vi "img test14(coutsegment attempt3).vi"() -> ()   [LabVIEW 2014]
uses:
  <vilib>/vision/NI_Vision_Development_Module.lvlib
panel:
  out "Array":dbl[][](array[numeric])
  in  "fast forward":bool
  out "Bottom Full movement patterns":string[](array[string])
  out "Top Full movement patterns":string[](array[string])
  out "bottom player pattern count 2":i32[](array[numeric])
  out "bottom player patterns 2":string[](array[string])
  out "top player pattern count":i32[](array[numeric])
  out "Top player patterns":string[](array[string])
  out "start":i32[](array[numeric])
  out "end":i32[](array[numeric])
  out "Infered action indicators":string[][](array[string])
  out "Movement data from both players":i32[][](array[numeric])
  out "end":i32[](array[numeric])
  out "start":i32[](array[numeric])
  in  "start":bool
  in  "End":bool
  in  "output array 4":string[][](array[string])
  in  "output array 3":string[][](array[string])
  in  "output array 2":string[][](array[string])=array2129x6[12774 elements]
  out "BOTTOM":string[](array[string])
  out "TOP":string[](array[string])
  in  "output array":string[][](array[string])=array1935x6[11610 elements]
  out "Number of Frames":u32
  out "Top player court segment display 2":bool[][](array[boolean])
  out "count top":i32[](graph)
  out "count bottom":i32[](graph)
  out "trans top":i32[](graph)
  out "trans bottom":i32[](graph)
  in  "ON":bool
  out "Top player court segment display":bool[][](array[boolean])
  out "bottom player":cluster{"Numeric":dbl, "Numeric":dbl}[](array[cluster])
  out "top player":cluster{"Numeric":dbl, "Numeric":dbl}[](array[cluster])
  in  "playing":bool
  out "Top VIew":cluster{"Numeric":dbl, "Numeric":dbl}[](graph)
  out "Image 4":T1(plugin-control)
  in  "frame jump":i32=3
  in  "speed":u32(slide)
  in  "start":i32(slide) step=219843704 scale=0.0..66731.0
  out "Image 3":T1(plugin-control)
  in  "AVI Path":path=path "E:/PhD work/PhD research work/Videos/Chen Jin vs Hu Yun (Edited).avi"
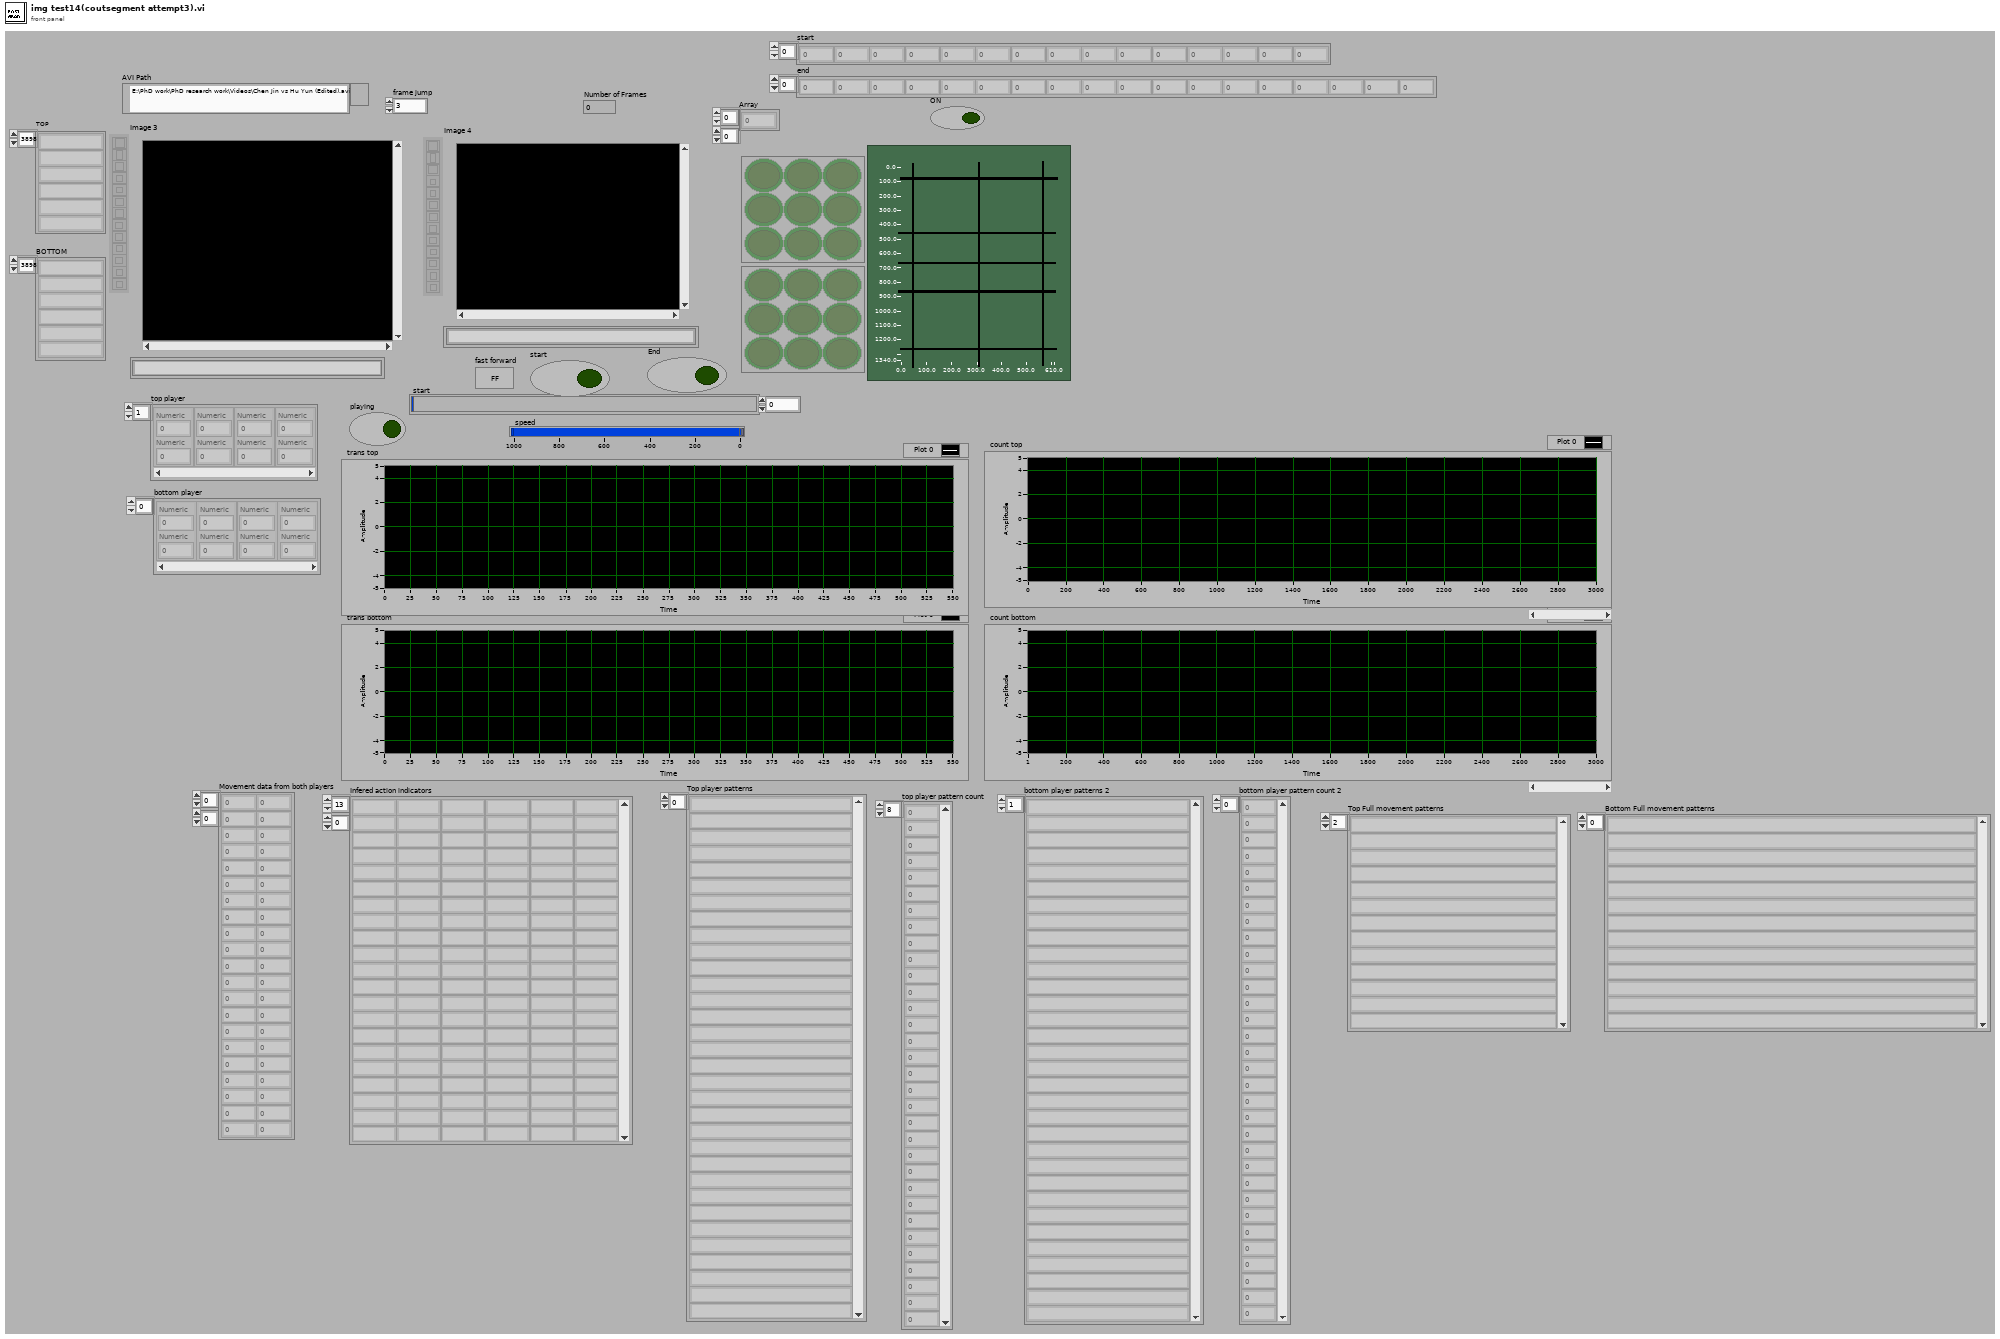
[diagram p1: front panel]
types:
  T1 = typedef "IMAQ Image.ctl" = refnum<image>
  T2 = cluster{cluster{"X":sgl, "Y":sgl}[], cluster{i32, i32}[], "Unit":u32}
  T3 = typedef "Image Type" = u32
  T4 = typedef "AviRefnum.ctl" = refnum<k1>
  T5 = cluster{"width":u32, "height":u32, "framesPerSecond":u32, "compressionFilter":string, "hasData":bool}
  T6 = cluster{"Origin Pixel":cluster{"X":sgl, "Y":sgl}, "Angle Relative to Horizontal (deg)":sgl, "Axis Reference":u32}
  T7 = typedef "Particle Parameters" = i32
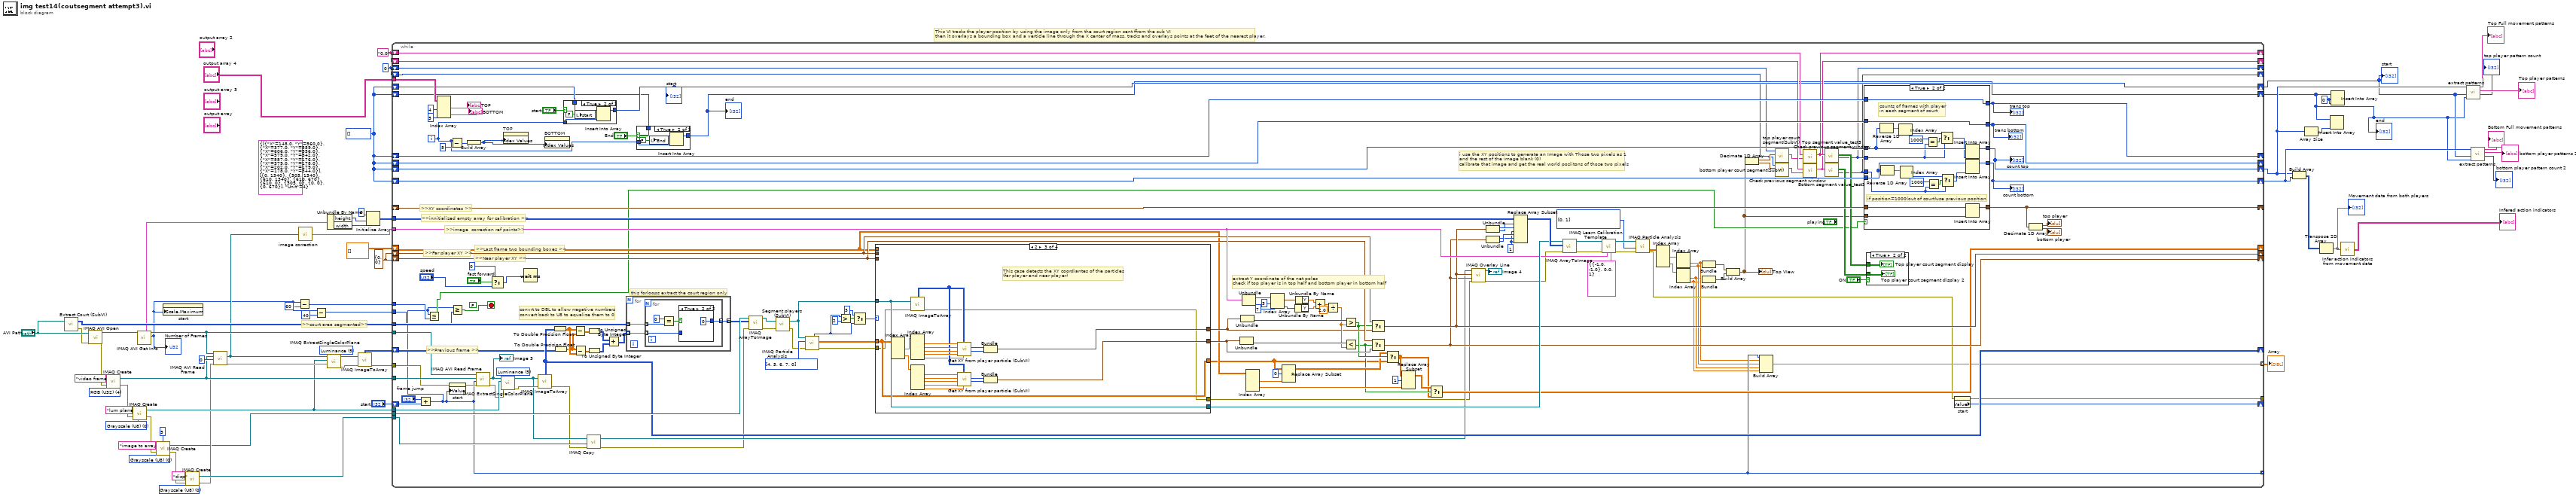
[diagram p0: block diagram]
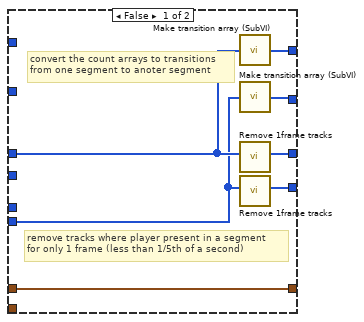
[diagram p4: hidden frame]
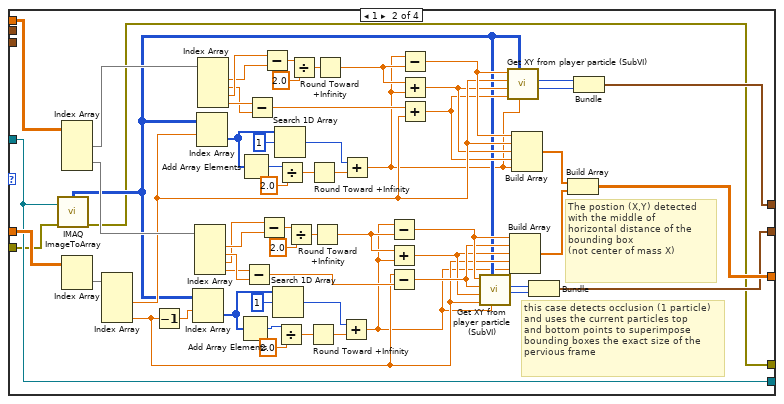
[diagram p7: hidden frame]
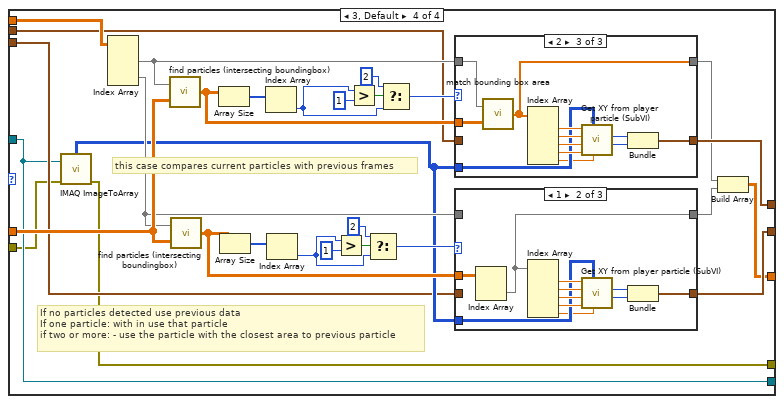
[diagram p8: hidden frame]
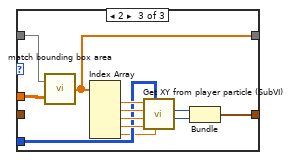
[diagram p10: hidden frame]
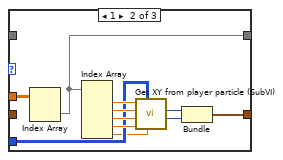
[diagram p12: hidden frame]
diagram:
  w2 = 0 ("Top player segment value")
  w14 = 0 ("index")
  (unwired) T2 {[{"X"=148.0, "Y"=560.0}, {"X"=377.0, "Y"=559.0}, {"X"=606.0, "Y"=556.0}, {"X"=579.0, "Y"=342.0}, {"X"=557.0, "Y"=176.0}, {"X"=379.0, "Y"=178.0}, {"X"=202.0, "Y"=179.0}, {"X"=178.0, "Y"=344.0}], [{0, 1340}, {305, 1340}, {610, 1340}, {610, 670}, {610, 0}, {305, 0}, {0, 0}, {0, 670}], "Unit"=4} ("ref points")
  w27 = "0,0" ("Player segment position")
  w18 = i32[] [] ("input array")
  w37 = cluster{"X coordinate":i32, "Y coordinate":i32} {"X coordinate"=0, "Y coordinate"=0}
  w50 = T3 0 items=["Grayscale (U8)", "Grayscale (I16)", "Grayscale (SGL)", "Complex (CSG)", "RGB (U32)", "HSL (U32)", "RGB (U64)", "Grayscale (U16)"] ("Image Type")
  w57 = 5 items=["Red", "Green", "Blue", "Hue", "Saturation", "Luminance", "Value", "Intensity"] ("Color Plane")
  w58 = T3 0 items=["Grayscale (U8)", "Grayscale (I16)", "Grayscale (SGL)", "Complex (CSG)", "RGB (U32)", "HSL (U32)", "RGB (U64)", "Grayscale (U16)"] ("Image Type")
  w62 = T3 0 items=["Grayscale (U8)", "Grayscale (I16)", "Grayscale (SGL)", "Complex (CSG)", "RGB (U32)", "HSL (U32)", "RGB (U64)", "Grayscale (U16)"] ("Image Type")
  w60 = T3 4 items=["Grayscale (U8)", "Grayscale (I16)", "Grayscale (SGL)", "Complex (CSG)", "RGB (U32)", "HSL (U32)", "RGB (U64)", "Grayscale (U16)"] ("Image Type")
  # ">>court area segmented>>"
  # "This VI tracks the player position by using the image only from the court region sent ffrom the sub VI\nthen it overlays a bounding box and a verticle line through the X center of mass. tracks and overlays points at the feet of the nearest player."
  n1 = call "Extract Court (SubVI).vi"("AVI Path"="AVI Path") -> ("error out"=w64:errorcluster, "Court pixels out"=w40:u8[][])  [unwired: 1 in]
  n2 = call "IMAQ AVI Open"("error in (no error)"=w64, "AVI Path"="AVI Path") -> ("error out"=w46:errorcluster, "Avi Refnum"=w35:T4)  [unwired: 8 in]
  n3 = call "IMAQ Create"("Image Name"="video frame", "Image Type"=w60, "error in (no error)"=w46) -> ("New Image"=w54:T1, "error out"=w45:errorcluster)  [unwired: 2 in]
  n4 = call "IMAQ Create"("Image Name"="lum plane", "Image Type"=w62, "error in (no error)"=w45) -> ("New Image"=w53:T1, "error out"=w44:errorcluster)  [unwired: 2 in]
  n5 = call "IMAQ AVI Get Info"("Avi Refnum"=w35) -> ("Number of Frames"=w25:u32, "Avi Refnum (duplicate)"=w34:T4, "Frame Data"=w31:T5)  [unwired: 6 in, 2 out]
  "Number of Frames" <- w25
  n6 = call "IMAQ Create"("Border Size"=5, "Image Name"="image to array", "Image Type"=w58, "error in (no error)"=w44) -> ("New Image"=w39:T1, "error out"=w43:errorcluster)  [unwired: 1 in]
  n7 = property on="start" class="Slide (strict)"("Scale.Maximum"=w25) -> ()  [unwired: 2 in, 2 out]
  n8 = call "IMAQ Create"("Image Name"="disp", "Image Type"=w50, "error in (no error)"=w43) -> ("New Image"=w48:T1, "error out"=w42:errorcluster)  [unwired: 2 in]
  n9 = call "IMAQ AVI Read Frame"("error in (no error)"=w42, "Frame Number"=u32 0, "Image"=w54, "Avi Refnum"=w34) -> ("error out"=w56:errorcluster, "Image Out"=w26:T1)  [unwired: 4 in, 2 out]
  n10 = Subtract(x=w25, y=u32 60) -> (x-y=w22:u32)
  n11 = call "image correction.vi"("Image"=w26) -> ("ref points"=w20:T2)
  n12 = Subtract(x=w25, y=u32 40) -> (x-y=w21:u32)
  n13 = Unbundle By Name(w31) -> ("height"=w30:u32, "width"=w29:u32)
  n14 = call "IMAQ ExtractSingleColorPlane"("Color Plane"=w57, "error in (no error)"=w56, "Image Dst"=w53, "Image Src"=w26) -> ("error out"=w47:errorcluster, "Image Dst Out"=w51:T1)  [unwired: 6 in]
  n15 = call "IMAQ ImageToArray"("error in (no error)"=w47, "Image"=w51) -> ("error out"=w33:errorcluster, "Image Pixels (U8)"=w52:u8[][])  [unwired: 2 in, 3 out]
  n16 = Initialize Array(u8 0 ("element"), w30, w29) -> (w28:u8[][])
  n17 = while {
    tunnel: w34 -> [w187]
    tunnel: w54 -> [w204]
    tunnel: w40 -> [w217]
    tunnel: w53 -> [w205]
    tunnel: w39 -> [w216]
    shift-right: [w215] -> _
    shift-left: w52 -> [w214]
    tunnel: w48 -> [w190]
    shift-right: [w133] -> _
    shift-left: dbl[][] [] ("Particle Measurements (Pixels)") -> [w143]
    shift-right: [w147] -> _
    shift-left: w37 -> [w149]
    shift-right: [w145] -> _
    shift-left: w37 -> [w148]
    shift-right: [w184] -> _
    shift-left: "start" -> [w189]
    tunnel: w33 -> [w186]
    tunnel: w28 -> [w183]
    tunnel: w20 -> [w162]
    shift-right: [w117] -> _
    shift-left: _ -> [w166]
    shift-right: [w92] -> w12
    shift-left: w18 -> [w120]
    shift-right: [w93] -> w11
    shift-left: w18 -> [w121]
    tunnel: [w123] -> _
    shift-right: [w111] -> _
    shift-left: w18 -> [w118]
    shift-right: [w116] -> _
    shift-left: w18 -> [w119]
    shift-right: [w105] -> _
    shift-left: w27 -> [w112]
    shift-right: [w106] -> _
    shift-left: w27 -> [w113]
    tunnel: w22 -> [w104]
    tunnel: w21 -> [w103]
    tunnel: [w71] -> _ mode=indexing
    tunnel: "output array 4" -> [w98]
    shift-right: [w84] -> w3
    shift-left: w18 -> [w85]
    shift-right: [w86] -> w4
    shift-left: w18 -> [w87]
    shift-right: [w75] -> _
    shift-left: w2 -> [w73]
    shift-right: [w74] -> _
    shift-left: w2 -> [w72]
    tunnel: [w66] -> w1 mode=indexing
    i -> [w82]
    stop <- w110 stop-if-true
    w170 = T7[] [0, 1] items=["Center of Mass X", "Center of Mass Y", "First Pixel X", "First Pixel Y", "Bounding Rect Left", "Bounding Rect Top", "Bounding Rect Right", "Bounding Rect Bottom", "Max Feret Diameter Start X", "Max Feret Diameter Start Y", "Max Feret Diameter End X", "Max Feret Diameter End Y", "Max Horiz. Segment Length Left", "Max Horiz. Segment Length Right", "Max Horiz. Segment Length Row", "-", "Bounding Rect Width", "Bounding Rect Height", "Bounding Rect Diagonal", "Perimeter", "Convex Hull Perimeter", "Holes' Perimeter", "Max Feret Diameter", "Equivalent Ellipse Major Axis", "Equivalent Ellipse Minor Axis", "Equivalent Ellipse Minor Axis (Feret)", "Equivalent Rect Long Side", "Equivalent Rect Short Side", "Equivalent Rect Diagonal", "Equivalent Rect Short Side (Feret)", "Average Horiz. Segment Length", "Average Vert. Segment Length", "Hydraulic Radius", "Waddel Disk Diameter", "-", "Area", "Holes' Area", "Particle & Holes' Area", "Convex Hull Area", "Image Area", "-", "Number of Holes", "Number of Horiz. Segments", "Number of Vert. Segments", "-", "Orientation", "Max Feret Diameter Orientation", "-", "% Area/Image Area", "% Area/(Particle & Holes' Area)", "Ratio of Equivalent Ellipse Axes", "Ratio of Equivalent Rect Sides", "-", "Elongation Factor", "Compactness Factor", "Heywood Circularity Factor", "Type Factor", "-", "Sum X", "Sum Y", "Sum XX", "Sum XY", "Sum YY", "Sum XXX", "Sum XXY", "Sum XYY", "Sum YYY", "-", "Moment of Inertia XX", "Moment of Inertia XY", "Moment of Inertia YY", "Moment of Inertia XXX", "Moment of Inertia XXY", "Moment of Inertia XYY", "Moment of Inertia YYY", "Norm. Moment of Inertia XX", "Norm. Moment of Inertia XY", "Norm. Moment of Inertia YY", "Norm. Moment of Inertia XXX", "Norm. Moment of Inertia XXY", "Norm. Moment of Inertia XYY", "Norm. Moment of Inertia YYY", "Hu Moment 1", "Hu Moment 2", "Hu Moment 3", "Hu Moment 4", "Hu Moment 5", "Hu Moment 6", "Hu Moment 7"] ("Real-World Measurements")
    w178 = u8 1 ("new element/subarray")
    w206 = T7[] [4, 5, 6, 7, 0] items=["Center of Mass X", "Center of Mass Y", "First Pixel X", "First Pixel Y", "Bounding Rect Left", "Bounding Rect Top", "Bounding Rect Right", "Bounding Rect Bottom", "Max Feret Diameter Start X", "Max Feret Diameter Start Y", "Max Feret Diameter End X", "Max Feret Diameter End Y", "Max Horiz. Segment Length Left", "Max Horiz. Segment Length Right", "Max Horiz. Segment Length Row", "-", "Bounding Rect Width", "Bounding Rect Height", "Bounding Rect Diagonal", "Perimeter", "Convex Hull Perimeter", "Holes' Perimeter", "Max Feret Diameter", "Equivalent Ellipse Major Axis", "Equivalent Ellipse Minor Axis", "Equivalent Ellipse Minor Axis (Feret)", "Equivalent Rect Long Side", "Equivalent Rect Short Side", "Equivalent Rect Diagonal", "Equivalent Rect Short Side (Feret)", "Average Horiz. Segment Length", "Average Vert. Segment Length", "Hydraulic Radius", "Waddel Disk Diameter", "-", "Area", "Holes' Area", "Particle & Holes' Area", "Convex Hull Area", "Image Area", "-", "Number of Holes", "Number of Horiz. Segments", "Number of Vert. Segments", "-", "Orientation", "Max Feret Diameter Orientation", "-", "% Area/Image Area", "% Area/(Particle & Holes' Area)", "Ratio of Equivalent Ellipse Axes", "Ratio of Equivalent Rect Sides", "-", "Elongation Factor", "Compactness Factor", "Heywood Circularity Factor", "Type Factor", "-", "Sum X", "Sum Y", "Sum XX", "Sum XY", "Sum YY", "Sum XXX", "Sum XXY", "Sum XYY", "Sum YYY", "-", "Moment of Inertia XX", "Moment of Inertia XY", "Moment of Inertia YY", "Moment of Inertia XXX", "Moment of Inertia XXY", "Moment of Inertia XYY", "Moment of Inertia YYY", "Norm. Moment of Inertia XX", "Norm. Moment of Inertia XY", "Norm. Moment of Inertia YY", "Norm. Moment of Inertia XXX", "Norm. Moment of Inertia XXY", "Norm. Moment of Inertia XYY", "Norm. Moment of Inertia YYY", "Hu Moment 1", "Hu Moment 2", "Hu Moment 3", "Hu Moment 4", "Hu Moment 5", "Hu Moment 6", "Hu Moment 7"] ("Pixel Measurements")
    (unwired) FALSE
    w218 = 5 items=["Red", "Green", "Blue", "Hue", "Saturation", "Luminance", "Value", "Intensity"] ("Color Plane")
    # ">>XY coordinates >>"
    # ">>innitialized empty array for calibration >>"
    # ">>image  correction ref points>>"
    # "extract Y coordinate of the net poles\ncheck if top player is in top half and bottom player in bottom half"
    # "i use the XY positions to generate an Image with Those two pixels as 1 \nand the rest of the image blank (0)\ncalibrate that image and get the real world posiitons of those two pixels"
    # ">>Last frame two bounding boxes >>"
    # ">>Far player XY >>"
    # ">>Near player XY >>"
    # ">>Previous frame >>"
    # "convrt to DBL to allow negative numbers\nconvert back to U8 to equalize them to 0"
    # "this forloops extract the court region only"
    n18 = Add(x="frame jump", y=w189) -> (x+y=w71:i32)
    n19 = Less Or Equal?(x=w71, y=w104) -> (x <= y?=w109:bool)
    n20 = Index Array(array=w98, index (col) #1=4 ("disabled index (col)"), index (col) #2=5 ("index (col)")) -> (element #1=→"TOP":string[], element #2=→"BOTTOM":string[])  [unwired: 2 in]
    n21 = property on="start" class="Slide (strict)"(error in=w186, "Value"=w71) -> (error out=w185:errorcluster)  [unwired: 1 in, 1 out]
    n22 = Subtract(x=w82, y=5) -> (x-y=w90:i32)
    n23 = Greater Or Equal?(x=w71, y=w103) -> (x >= y?=w110:bool)
    n24 = Build Array(w90) -> (w89:i32[])
    n25 = call "IMAQ AVI Read Frame"("error in (no error)"=w185, "Frame Number"=w71, "Image"=w204, "Avi Refnum"=w187) -> ("error out"=w99:errorcluster, "Image Out"=w102:T1)  [unwired: 4 in, 2 out]
    "Image 3" <- w102
    n26 = Select(t=u32 0, s="fast forward", f="speed") -> (s? t:f=w77:u32)
    n27 = call "IMAQ ExtractSingleColorPlane"("Color Plane"=w218, "error in (no error)"=w99, "Image Dst"=w205, "Image Src"=w102) -> ("error out"=w207:errorcluster, "Image Dst Out"=w191:T1)  [unwired: 6 in]
    n28 = property on="TOP" class="Arr (strict)"("Index Values"=w89) -> ()  [unwired: 2 in, 2 out]
    n29 = Wait (ms)(milliseconds to wait=w77) -> ()  [unwired: 1 out]
    n30 = call "IMAQ ImageToArray"("error in (no error)"=w207, "Image"=w191) -> ("error out"=w128:errorcluster, "Image Pixels (U8)"=w215:u8[][])  [unwired: 2 in, 3 out]
    n31 = property on="BOTTOM" class="Arr (strict)"("Index Values"=w89) -> ()  [unwired: 2 in, 2 out]
    n32 = To Double Precision Float(number=w215) -> (double precision float=w211:dbl[][])
    n33 = To Double Precision Float(number=w214) -> (double precision float=w210:dbl[][])
    n34 = case shown="True" "start" {
      tunnel: w87 -> [w224 w228]
      tunnel: w82 -> [_ w227]
      tunnel: [w224 w226] -> w86
      frame False {
      }
      frame True {
        n35 = local write "start"(FALSE ("start")) -> ()
        n36 = Insert Into Array(array=w228, new element=w227) -> (w226:i32[])  [unwired: 1 in]
      }
    }
    "start" <- w86
    n37 = Subtract(x=w211, y=w210) -> (x-y=w209:dbl[][])
    n38 = Subtract(x=w210, y=w211) -> (x-y=w208:dbl[][])
    n39 = call "IMAQ Copy"("error in (no error)"=w128, "Image Dst"=w190, "Image Src"=w191) -> ("error out"=w127:errorcluster, "Image Dst Out"=w129:T1)  [unwired: 3 in]
    n40 = To Unsigned Byte Integer(number=w209) -> (unsigned 8bit integer=w213:u8[][])
    n41 = To Unsigned Byte Integer(number=w208) -> (unsigned 8bit integer=w212:u8[][])
    n42 = Add(x=w213, y=w212) -> (x+y=w81:u8[][])
    n43 = for {
      tunnel: w217 -> [w429] mode=indexing
      tunnel: [w428] -> w80 mode=indexing
      tunnel: w81 -> [w427] mode=indexing
      n44 = for {
        tunnel: w429 -> [w434] mode=indexing
        tunnel: [w431] -> w428 mode=indexing
        tunnel: w427 -> [w430] mode=indexing
        n45 = Equal?(x=u8 0, y=w434) -> (x = y?=w432:bool)
        n46 = case shown="True" w432 {
          tunnel: [w435 u8 0 ("x")] -> w431
          tunnel: w430 -> [w435 _]
          frame False {
          }
          frame True {
          }
        }
      }
    }
    n47 = case shown="True" "End" {
      tunnel: w85 -> [w219 w223]
      tunnel: w82 -> [_ w222]
      tunnel: [w219 w221] -> w84
      frame False {
      }
      frame True {
        n48 = local write "End"(FALSE ("End")) -> ()
        n49 = Insert Into Array(array=w223, new element=w222) -> (w221:i32[])  [unwired: 1 in]
      }
    }
    "end" <- w84
    n50 = call "IMAQ ArrayToImage"("error in (no error)"=w127, "Image Pixels (U8)"=w80, "Image"=w216) -> ("error out"=w202:errorcluster, "Image Out"=w203:T1)  [unwired: 7 in]
    n51 = call "Segment players (SubVI).vi"("error In"=w202, "Image In"=w203) -> ("error out"=w196:errorcluster, "Image Out"=w194:T1)
    n52 = call "IMAQ Particle Analysis"("error in (no error)"=w196, "Pixel Measurements"=w206, "Image"=w194) -> ("error out"=w195:errorcluster, "Particle Measurements (Pixels)"=w193:dbl[][], "Number of Particles"=w198:i32)  [unwired: 3 in, 3 out]
    n53 = Greater?(x=w198, y=2) -> (0:w201:bool)
    n54 = Select(t=3 ("y"), s=w201, f=w198) -> (s? t:f=w197:i32)
    n55 = case shown="2" w197 {
      tunnel: [w262 w289 w343 w353] -> w176
      tunnel: w193 -> [_ w324 w329 w373]
      tunnel: w195 -> [w259 w265 w326 w349]
      tunnel: w194 -> [w262 w289 w343 w353]
      tunnel: [w260 w273 w331 w355] -> w144
      tunnel: [w261 w280 w330 w354] -> w146
      tunnel: [w263 w290 w329 w350] -> w132
      tunnel: w143 -> [w263 w314 _ w376]
      tunnel: w149 -> [w261 _ _ w361]
      tunnel: w148 -> [w260 _ _ w356]
      tunnel: [w259 w264 w325 w348] -> w125
      frame 0 {
        # "This case identifies frames where no particles are detected and keeps the same values from the\nprevious frame"
      }
      frame 1 {
        # "The postion (X,Y) detected with the middle of \nhorizontal distance of the bounding box\n(not center of mass X)"
        # "this case detects occlusion (1 particle)\nand uses the current particles top \nand bottom points to superimpose \nbounding boxes the exact size of the \npervious frame"
        n56 = call "IMAQ ImageToArray"("error in (no error)"=w265, "Image"=w289) -> ("error out"=w264:errorcluster, "Image Pixels (U8)"=w272:u8[][])  [unwired: 2 in, 3 out]
        n57 = Index Array(array=w314) -> (element #1=w322:dbl[], element #2=w294:dbl[])  [unwired: 4 in]
        n58 = Index Array(array=w324) -> (element=w323:dbl[])  [unwired: 2 in]
        n59 = Index Array(array=w323) -> (element #2=w285:dbl, element #4=w276:dbl)  [unwired: 4 in, 2 out]
        n60 = Decrement(x=w276) -> (x-1=w287:dbl)
        n61 = Index Array(array=w272, index (row)=w287) -> (element=w309:u8[])  [unwired: 1 in]
        n62 = Index Array(array=w294) -> (element #1=w298:dbl, element #2=w301:dbl, element #3=w297:dbl, element #4=w300:dbl)  [unwired: 4 in]
        n63 = Index Array(array=w272, index (row)=w285) -> (element=w302:u8[])  [unwired: 1 in]
        n64 = Index Array(array=w322) -> (element #1=w318:dbl, element #2=w315:dbl, element #3=w319:dbl, element #4=w316:dbl)  [unwired: 4 in]
        n65 = Add Array Elements(numeric array=w309) -> (sum=w310:u8)
        n66 = Add Array Elements(numeric array=w302) -> (sum=w306:u8)
        n67 = Subtract(x=w300, y=w301) -> (x-y=w288:dbl)
        n68 = Subtract(x=w316, y=w315) -> (x-y=w293:dbl)
        n69 = Subtract(x=w297, y=w298) -> (x-y=w296:dbl)
        n70 = Subtract(x=w319, y=w318) -> (x-y=w320:dbl)
        n71 = Search 1D Array(1D array=w309, element=u8 1) -> (index of element=w308:i32)  [unwired: 1 in]
        n72 = Search 1D Array(1D array=w302, element=u8 1) -> (index of element=w307:i32)  [unwired: 1 in]
        n73 = Divide(x=w310, y=2.0) -> (x/y=w311:dbl)
        n74 = Divide(x=w306, y=2.0) -> (x/y=w305:dbl)
        n75 = Divide(x=w296, y=2.0) -> (x/y=w299:dbl)
        n76 = Divide(x=w320, y=2.0) -> (x/y=w317:dbl)
        n77 = Round Toward +Infinity(x=w311) -> (ceil(x): smallest int >= x=w270:dbl)
        n78 = Round Toward +Infinity(x=w305) -> (ceil(x): smallest int >= x=w269:dbl)
        n79 = Round Toward +Infinity(x=w299) -> (ceil(x): smallest int >= x=w271:dbl)
        n80 = Round Toward +Infinity(x=w317) -> (ceil(x): smallest int >= x=w268:dbl)
        n81 = Add(x=w308, y=w270) -> (x+y=w266:dbl)
        n82 = Add(x=w307, y=w269) -> (x+y=w267:dbl)
        n83 = Subtract(x=w266, y=w271) -> (x-y=w279:dbl)
        n84 = Add(x=w271, y=w266) -> (x+y=w277:dbl)
        n85 = Subtract(x=w276, y=w288) -> (x-y=w278:dbl)
        n86 = Subtract(x=w267, y=w268) -> (x-y=w286:dbl)
        n87 = Add(x=w268, y=w267) -> (x+y=w284:dbl)
        n88 = Add(x=w293, y=w285) -> (x+y=w283:dbl)
        n89 = call "Get XY from player particle (SubVI).vi"("Center of mass X"=w266, "Image in Pixels (U8)"=w272, "Particle bounding rect bottom"=w276, "Particle bounding rect right"=w277, "Particle bounding rect top"=w278, "Particle bounding rect left"=w279) -> ("Y coordinate"=w274:i32, "X coordinate"=w275:i32)  [unwired: 2 in]
        n90 = call "Get XY from player particle (SubVI).vi"("Center of mass X"=w267, "Image in Pixels (U8)"=w272, "Particle bounding rect bottom"=w283, "Particle bounding rect right"=w284, "Particle bounding rect top"=w285, "Particle bounding rect left"=w286) -> ("Y coordinate"=w281:i32, "X coordinate"=w282:i32)  [unwired: 2 in]
        n91 = Build Array(w279, w278, w277, w276, w266) -> (w291:dbl[])
        n92 = Build Array(w286, w285, w284, w283, w267) -> (w292:dbl[])
        n93 = Bundle("X coordinate"=w275, "Y coordinate"=w274) -> (w273:cluster{"X coordinate":i32, "Y coordinate":i32})  [unwired: 1 in]
        n94 = Build Array(w292, w291) -> (w290:dbl[][])
        n95 = Bundle("X coordinate"=w282, "Y coordinate"=w281) -> (w280:cluster{"X coordinate":i32, "Y coordinate":i32})  [unwired: 1 in]
      }
      frame 2 {
        # "This case detects the XY coordiantes of the particles\n(far player and near player)"
        n96 = Index Array(array=w329) -> (element #1=w337:dbl[], element #2=w336:dbl[])  [unwired: 4 in]
        n97 = call "IMAQ ImageToArray"("error in (no error)"=w326, "Image"=w343) -> ("error out"=w325:errorcluster, "Image Pixels (U8)"=w338:u8[][])  [unwired: 2 in, 3 out]
        n98 = Index Array(array=w337) -> (element #1=w347:dbl, element #2=w346:dbl, element #3=w345:dbl, element #4=w344:dbl, element #5=w328:dbl)  [unwired: 5 in]
        n99 = Index Array(array=w336) -> (element #1=w339:dbl, element #2=w340:dbl, element #3=w341:dbl, element #4=w342:dbl, element #5=w327:dbl)  [unwired: 5 in]
        n100 = call "Get XY from player particle (SubVI).vi"("Center of mass X"=w328, "Image in Pixels (U8)"=w338, "Particle bounding rect bottom"=w344, "Particle bounding rect right"=w345, "Particle bounding rect top"=w346, "Particle bounding rect left"=w347) -> ("Y coordinate"=w334:i32, "X coordinate"=w335:i32)  [unwired: 2 in]
        n101 = call "Get XY from player particle (SubVI).vi"("Center of mass X"=w327, "Image in Pixels (U8)"=w338, "Particle bounding rect bottom"=w342, "Particle bounding rect right"=w341, "Particle bounding rect top"=w340, "Particle bounding rect left"=w339) -> ("Y coordinate"=w332:i32, "X coordinate"=w333:i32)  [unwired: 2 in]
        n102 = Bundle("X coordinate"=w335, "Y coordinate"=w334) -> (w330:cluster{"X coordinate":i32, "Y coordinate":i32})  [unwired: 1 in]
        n103 = Bundle("X coordinate"=w333, "Y coordinate"=w332) -> (w331:cluster{"X coordinate":i32, "Y coordinate":i32})  [unwired: 1 in]
      }
      frame 3, Default {
        # "If no particles detected use previous data\nIf one particle: with in use that particle\nif two or more: - use the particle with the closest area to previous particle"
        # "this case compares current particles with previous frames"
        n104 = call "IMAQ ImageToArray"("error in (no error)"=w349, "Image"=w353) -> ("error out"=w348:errorcluster, "Image Pixels (U8)"=w357:u8[][])  [unwired: 2 in, 3 out]
        n105 = Index Array(array=w376) -> (element #1=w372:dbl[], element #2=w360:dbl[])  [unwired: 4 in]
        n106 = call "find particles (intersecting boundingbox).vi"("Particle Measurements in (bounding boxes)"=w373, "bounding box in"=w372) -> ("Particles within bounding box"=w371:dbl[][])
        n107 = call "find particles (intersecting boundingbox).vi"("Particle Measurements in (bounding boxes)"=w373, "bounding box in"=w360) -> ("Particles within bounding box"=w358:dbl[][])
        n108 = Array Size(array=w371) -> (size(s)=w375:i32[])
        n109 = Array Size(array=w358) -> (size(s)=w374:i32[])
        n110 = Index Array(array=w375) -> (element=w363:i32)  [unwired: 1 in]
        n111 = Index Array(array=w374) -> (element=w364:i32)  [unwired: 1 in]
        n112 = Greater?(x=w364, y=1) -> (0:w367:bool)
        n113 = Greater?(x=w363, y=1) -> (0:w368:bool)
        n114 = Select(t=2 ("y"), s=w367, f=w364) -> (s? t:f=w359:i32)
        n115 = Select(t=2 ("y"), s=w368, f=w363) -> (s? t:f=w362:i32)
        n116 = case shown="2" w362 {
          tunnel: w372 -> [w403 _ w418]
          tunnel: w371 -> [_ w414 w417]
          tunnel: [w403 w405 w416] -> w352
          tunnel: w357 -> [_ w407 w420]
          tunnel: [w402 w406 w419] -> w354
          tunnel: w361 -> [w402 _ _]
          frame 0, Default {
          }
          frame 1 {
            n117 = Index Array(array=w414) -> (element=w405:dbl[])  [unwired: 2 in]
            n118 = Index Array(array=w405) -> (element #1=w411:dbl, element #2=w410:dbl, element #3=w409:dbl, element #4=w408:dbl, element #5=w404:dbl)  [unwired: 5 in]
            n119 = call "Get XY from player particle (SubVI).vi"("Center of mass X"=w404, "Image in Pixels (U8)"=w407, "Particle bounding rect bottom"=w408, "Particle bounding rect right"=w409, "Particle bounding rect top"=w410, "Particle bounding rect left"=w411) -> ("Y coordinate"=w412:i32, "X coordinate"=w413:i32)  [unwired: 2 in]
            n120 = Bundle("X coordinate"=w413, "Y coordinate"=w412) -> (w406:cluster{"X coordinate":i32, "Y coordinate":i32})  [unwired: 1 in]
          }
          frame 2 {
            n121 = call "match bounding box area.vi"("particle measurements (bounding box)"=w417, "bounding box in"=w418) -> ("matching bounding box"=w416:dbl[])
            n122 = Index Array(array=w416) -> (element #1=w424:dbl, element #2=w423:dbl, element #3=w422:dbl, element #4=w421:dbl, element #5=w415:dbl)  [unwired: 5 in]
            n123 = call "Get XY from player particle (SubVI).vi"("Center of mass X"=w415, "Image in Pixels (U8)"=w420, "Particle bounding rect bottom"=w421, "Particle bounding rect right"=w422, "Particle bounding rect top"=w423, "Particle bounding rect left"=w424) -> ("Y coordinate"=w425:i32, "X coordinate"=w426:i32)  [unwired: 2 in]
            n124 = Bundle("X coordinate"=w426, "Y coordinate"=w425) -> (w419:cluster{"X coordinate":i32, "Y coordinate":i32})  [unwired: 1 in]
          }
        }
        n125 = case shown="1" w359 {
          tunnel: w360 -> [w378 _ w393]
          tunnel: w358 -> [_ w389 w392]
          tunnel: [w378 w380 w391] -> w351
          tunnel: w357 -> [_ w382 w395]
          tunnel: [w377 w381 w394] -> w355
          tunnel: w356 -> [w377 _ _]
          frame 0, Default {
          }
          frame 1 {
            n126 = Index Array(array=w389) -> (element=w380:dbl[])  [unwired: 2 in]
            n127 = Index Array(array=w380) -> (element #1=w386:dbl, element #2=w385:dbl, element #3=w384:dbl, element #4=w383:dbl, element #5=w379:dbl)  [unwired: 5 in]
            n128 = call "Get XY from player particle (SubVI).vi"("Center of mass X"=w379, "Image in Pixels (U8)"=w382, "Particle bounding rect bottom"=w383, "Particle bounding rect right"=w384, "Particle bounding rect top"=w385, "Particle bounding rect left"=w386) -> ("Y coordinate"=w387:i32, "X coordinate"=w388:i32)  [unwired: 2 in]
            n129 = Bundle("X coordinate"=w388, "Y coordinate"=w387) -> (w381:cluster{"X coordinate":i32, "Y coordinate":i32})  [unwired: 1 in]
          }
          frame 2 {
            n130 = call "match bounding box area.vi"("particle measurements (bounding box)"=w392, "bounding box in"=w393) -> ("matching bounding box"=w391:dbl[])
            n131 = Index Array(array=w391) -> (element #1=w399:dbl, element #2=w398:dbl, element #3=w397:dbl, element #4=w396:dbl, element #5=w390:dbl)  [unwired: 5 in]
            n132 = call "Get XY from player particle (SubVI).vi"("Center of mass X"=w390, "Image in Pixels (U8)"=w395, "Particle bounding rect bottom"=w396, "Particle bounding rect right"=w397, "Particle bounding rect top"=w398, "Particle bounding rect left"=w399) -> ("Y coordinate"=w400:i32, "X coordinate"=w401:i32)  [unwired: 2 in]
            n133 = Bundle("X coordinate"=w401, "Y coordinate"=w400) -> (w394:cluster{"X coordinate":i32, "Y coordinate":i32})  [unwired: 1 in]
          }
        }
        n134 = Build Array(w352, w351) -> (w350:dbl[][])
      }
    }
    n135 = Unbundle(w144) -> ("Y coordinate"=w151:i32)  [unwired: 1 out]
    n136 = Unbundle(w146) -> ("Y coordinate"=w152:i32)  [unwired: 1 out]
    n137 = Unbundle(w162) -> (w161:cluster{"X":sgl, "Y":sgl}[])  [unwired: 2 out]
    n138 = Index Array(array=w143) -> (element #1=w141:dbl[], element #2=w137:dbl[])  [unwired: 4 in]
    n139 = Index Array(array=w161, index #1=3 ("index"), index #2=7 ("index")) -> (element #1=w158:cluster{"X":sgl, "Y":sgl}, element #2=w157:cluster{"X":sgl, "Y":sgl})
    n140 = Replace Array Subset(array=w132, new element=w141, index (row)=0) -> (w140:dbl[][])  [unwired: 1 in]
    n141 = Unbundle By Name(w157) -> ("Y"=w155:sgl)
    n142 = Unbundle By Name(w158) -> ("Y"=w156:sgl)
    n143 = Add(x=w156, y=w155) -> (x+y=w154:sgl)
    n144 = Divide(x=w154, y=sgl 2.0) -> (x/y=w150:sgl)
    n145 = Greater?(x=w152, y=w150) -> (0:w142:bool)
    n146 = Less?(x=w151, y=w150) -> (x < y?=w135:bool)
    n147 = Select(t=w149, s=w142, f=w146) -> (s? t:f=w147:cluster{"X coordinate":i32, "Y coordinate":i32})
    n148 = Select(t=w148, s=w135, f=w144) -> (s? t:f=w145:cluster{"X coordinate":i32, "Y coordinate":i32})
    n149 = Select(t=w140, s=w142, f=w132) -> (s? t:f=w134:dbl[][])
    n150 = Replace Array Subset(array=w134, new element=w137, index (row)=1) -> (w136:dbl[][])  [unwired: 1 in]
    n151 = Select(t=w136, s=w135, f=w134) -> (s? t:f=w133:dbl[][])
    n152 = call "IMAQ Overlay Line"("error in (no error)"=w125, "End Point"=w145, "Start Point"=w147, "Image"=w129) -> ("error out"=w126:errorcluster, "Image Out"=→"Image 4":T1)  [unwired: 6 in]
    n153 = Unbundle(w145) -> ("X coordinate"=w179:i32, "Y coordinate"=w180:i32)
    n154 = Unbundle(w147) -> ("X coordinate"=w182:i32, "Y coordinate"=w181:i32)
    n155 = Replace Array Subset(array=w183, new element #1=w178, index (row) #1=w181, index (col) #1=w182, new element #2=w178, index (row) #2=w180, index (col) #2=w179) -> (w177:u8[][])
    n156 = call "IMAQ ArrayToImage"("error in (no error)"=w126, "Image Pixels (U8)"=w177, "Image"=w176) -> ("error out"=w173:errorcluster, "Image Out"=w174:T1)  [unwired: 7 in]
    n157 = call "IMAQ Learn Calibration Template"("Calibration Axis Info"=T6 {"Origin Pixel"={"X"=-1.0, "Y"=-1.0}, "Angle Relative to Horizontal (deg)"=0.0, "Axis Reference"=1}, "Reference Points"=w162, "error in (no error)"=w173, "Image"=w174) -> ("error out"=w172:errorcluster, "Calibrated Image"=w171:T1)  [unwired: 5 in, 1 out]
    n158 = call "IMAQ Particle Analysis"("error in (no error)"=w172, "Real-World Measurements"=w170, "Image"=w171) -> ("error out"=w124:errorcluster, "Particle Measurements (Real-World)"=w169:dbl[][])  [unwired: 3 in, 4 out]
    n159 = Index Array(array=w169) -> (element #1=w168:dbl[], element #2=w167:dbl[])  [unwired: 4 in]
    n160 = Index Array(array=w168) -> (element #1=w70:dbl, element #2=w69:dbl)  [unwired: 2 in]
    n161 = Index Array(array=w167) -> (element #1=w68:dbl, element #2=w67:dbl)  [unwired: 2 in]
    n162 = Bundle("Numeric"=w70, "Numeric"=w69) -> (w165:cluster{"Numeric":dbl, "Numeric":dbl})  [unwired: 1 in]
    n163 = Bundle("Numeric"=w68, "Numeric"=w67) -> (w100:cluster{"Numeric":dbl, "Numeric":dbl})  [unwired: 1 in]
    n164 = Build Array(w165, w100) -> (w101:cluster{"Numeric":dbl, "Numeric":dbl}[])
    "Top VIew" <- w101
    n165 = Decimate 1D Array(w101) -> (w130:cluster{"Numeric":dbl, "Numeric":dbl}[], w131:cluster{"Numeric":dbl, "Numeric":dbl}[])
    n166 = Build Array(w71, w70, w69, w68, w67) -> (w66:dbl[])
    n167 = call "top player court segment(SubVI).vi"("Top player position"=w130, "previous segment"=w73) -> ("Top player segment position"=w108:string)  [unwired: 9 in]
    n168 = call "bottom player court segment(SubVI).vi"("Bottom player position"=w131, "previous segment"=w72) -> ("Bottom player segment position"=w107:string)  [unwired: 9 in]
    n169 = call "Check previous segment window.vi"("Current player segment position"=w108, "Previous player segment position"=w113) -> ("Player segment position"=w106:string)  [unwired: 9 in]
    n170 = call "Check previous segment window.vi"("Current player segment position"=w107, "Previous player segment position"=w112) -> ("Player segment position"=w105:string)  [unwired: 9 in]
    n171 = call "Top segment value_test3.vi"("Top player segment position"=w106) -> ("Top player segment value"=w75:i32, "Top player court segment display"=w115:bool[][])  [unwired: 9 in]
    n172 = call "Bottom segment value_test3.vi"("Bottom player segment position"=w105) -> ("Bottom player segment"=w74:i32, "Bottom player court segment display"=w114:bool[][])  [unwired: 9 in]
    n173 = case shown="True" w109 {
      tunnel: w166 -> [w235 w256]
      tunnel: w101 -> [_ w255]
      tunnel: w121 -> [w232 w249]
      tunnel: w120 -> [w231 w239]
      tunnel: [w233 w250] -> w111
      tunnel: [w234 w251] -> w116
      tunnel: w74 -> [_ w236]
      tunnel: w75 -> [_ w244]
      tunnel: w119 -> [_ w251]
      tunnel: w118 -> [_ w250]
      tunnel: [w230 w254] -> w92
      tunnel: [w229 w253] -> w93
      tunnel: [w235 w252] -> w117
      frame False {
        # "convert the count arrays to transitions \nfrom one segment to anoter segment"
        # "remove tracks where player present in a segment \nfor only 1 frame (less than 1/5th of a second)"
        n174 = call "Make transition array (SubVI).vi"("count array in"=w232) -> ("Transition array out"=w233:i32[])
        n175 = call "Make transition array (SubVI).vi"("count array in"=w231) -> ("Transition array out"=w234:i32[])
        n176 = call "Remove 1frame tracks.vi"("count array in"=w232) -> ("count array out"=w229:i32[])  [unwired: 10 in]
        n177 = call "Remove 1frame tracks.vi"("count array in"=w231) -> ("count array out"=w230:i32[])  [unwired: 10 in]
      }
      frame True {
        # "if position=1000(out of court)use previous position"
        # "counts of frames with player\nin each segment of court"
        n178 = Reverse 1D Array(array=w249) -> (reversed array=w248:i32[])
        n179 = Reverse 1D Array(array=w239) -> (reversed array=w238:i32[])
        n180 = Index Array(array=w248) -> (element=w245:i32)  [unwired: 1 in]
        n181 = Index Array(array=w238) -> (element=w242:i32)  [unwired: 1 in]
        n182 = Equal?(x=1000 ("y"), y=w244) -> (x = y?=w246:bool)
        n183 = Equal?(x=1000 ("y"), y=w236) -> (x = y?=w241:bool)
        n184 = Select(t=w245, s=w246, f=w244) -> (s? t:f=w243:i32)
        n185 = Select(t=w242, s=w241, f=w236) -> (s? t:f=w237:i32)
        n186 = Insert Into Array(array=w249, new element=w243) -> (w253:i32[])  [unwired: 1 in]
        n187 = Insert Into Array(array=w239, new element=w237) -> (w254:i32[])  [unwired: 1 in]
        n188 = Insert Into Array(array=w256, new element=w255) -> (w252:cluster{"Numeric":dbl, "Numeric":dbl}[])  [unwired: 1 in]
      }
    }
    "trans bottom" <- w116
    "trans top" <- w111
    "count bottom" <- w92
    "count top" <- w93
    n189 = case shown="True" "ON" {
      tunnel: w115 -> [_ w258]
      tunnel: w114 -> [_ w257]
      frame False {
      }
      frame True {
        "Top player court segment display" <- w258
        "Top player court segment display 2" <- w257
      }
    }
    n190 = property on="start" class="Slide (strict)"(error in=w124) -> (error out=w123:errorcluster, "Value"=w184:i32)  [unwired: 1 in, 1 out]
    n191 = Decimate 1D Array(w117) -> (→"top player":cluster{"Numeric":dbl, "Numeric":dbl}[], →"bottom player":cluster{"Numeric":dbl, "Numeric":dbl}[])
  }
  "end" <- w3
  "start" <- w4
  "Array" <- w1
  n192 = Build Array(w11, w12) -> (w17:i32[][])
  n193 = Array Size(array=w11) -> (size(s)=w13:i32)
  n194 = Transpose 2D Array(2D array=w17) -> (transposed array=w15:i32[][])
  "Movement data from both players" <- w15
  n195 = Insert Into Array(array=w3, new element=w13) -> ()  [unwired: 1 in, 1 out]
  n196 = Insert Into Array(array=w3, index=w14, new element=w14) -> ()  [unwired: 1 out]
  n197 = call "Infer action indicators from movement data.vi"("movement data from both players"=w15) -> ("Infered action indicators"=→"Infered action indicators":string[][])
  n198 = call "extract patterns.vi"("end points in"=w3, "Start points in"=w4, "player movement data"=w11) -> ("Sub pattern count"=→"top player pattern count":i32[], "Sub patterns"=→"Top player patterns":string[], "Full movement patterns"=→"Top Full movement patterns":string[])  [unwired: 6 in]
  n199 = call "extract patterns.vi"("end points in"=w3, "Start points in"=w4, "player movement data"=w12) -> ("Sub pattern count"=→"bottom player pattern count 2":i32[], "Sub patterns"=→"bottom player patterns 2":string[], "Full movement patterns"=→"Bottom Full movement patterns":string[])  [unwired: 6 in]
